vi "KeyboardController.vi"(8 "Manual Control Cluster":T1 {"Speed" scale=0.0..5.0}) -> (0 "Manual Control Cluster":T1 {"Speed" scale=0.0..5.0}, 1 "Extend":bool, 2 "Stop Button":bool, 3 "Retract":bool, 4 "Speed":dbl)   [LabVIEW 2021]
uses:
  <vilib>/event_ctls.llb/eventvkey.ctl
  <vilib>/event_ctls.llb/lveventtype.ctl
  <vilib>/event_ctls.llb/eventsource.ctl
  ManualConttrolCluster.ctl
panel:
  out "ScanCode":i16
  out "Time":u32
  out "PlatMods":T2
  out "Mods":cluster{"Num Pad":bool, "Menu Key":bool}
  out "Source":T3 items=["LabVIEW UI"=0, "ActiveX"=1, "User Event"=25]
  out "Type":T4=enum."Value Change"
  out "VKey":T5
  out "Char":i16
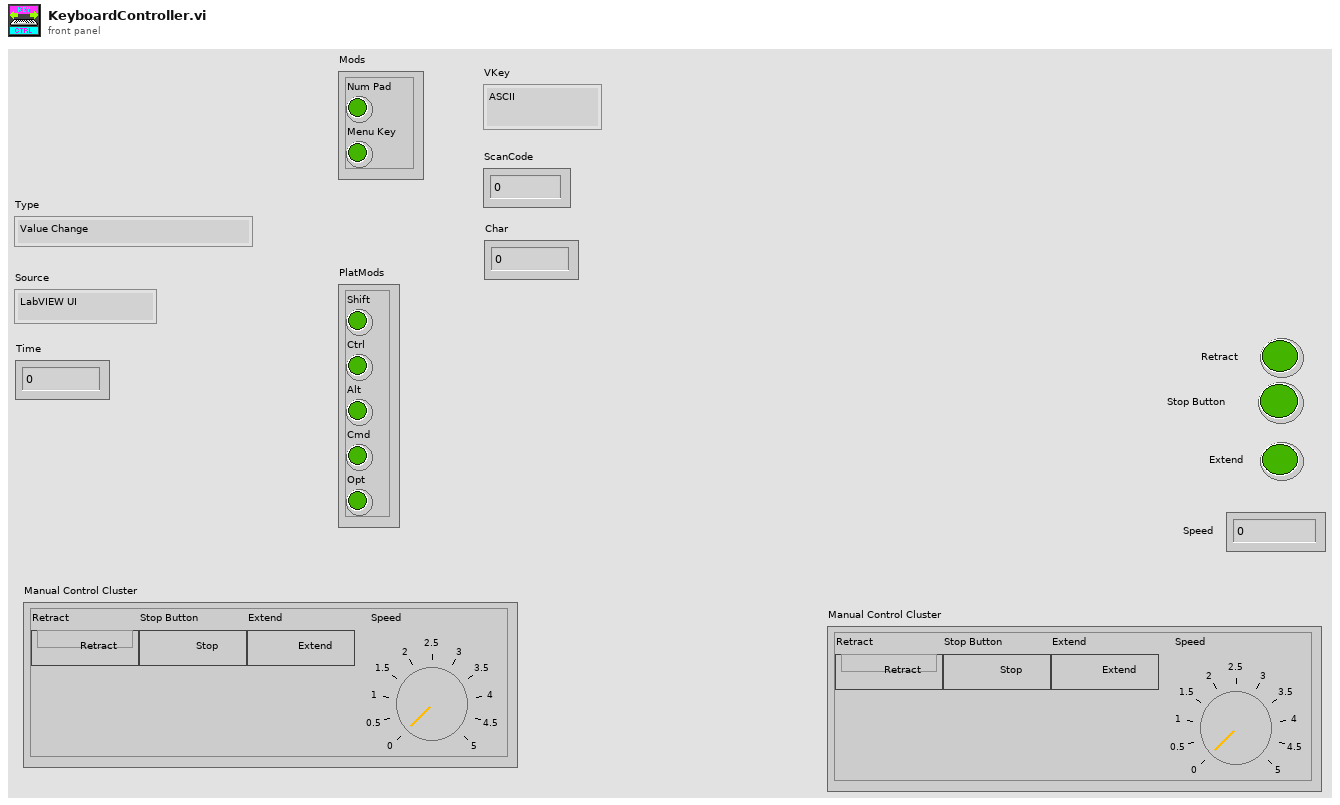
[diagram p1: front panel]
types:
  T1 = typedef "ManualConttrolCluster.ctl" = cluster{"Retract":bool, "Stop Button":bool, "Extend":bool, "Speed":dbl}
  T2 = cluster{"Shift":bool, "Ctrl":bool, "Alt":bool, "Cmd":bool, "Opt":bool}
  T3 = typedef "eventsource.ctl" = u32
  T4 = typedef "lveventtype.ctl" = enum32{"Null", "Timeout", "Annotation Menu Selection", "Annotation Menu Selection?", "App Instance Close", "App Instance Close?", "Autoscale Range Change", "Bookmark Info Change", "Cell Edit", "Cell Edit?", "Cursor Grab", "Cursor Grab?", "Cursor Menu Selection", "Cursor Menu Selection?", "Cursor Move", "Cursor Release", "Data Change", "Direction Change", "Display State Change", "Drag Ended", "Drag Enter", "Drag Leave", "Drag Over", "Drag Source Update", "Drag Starting", "Drag Starting?", "Drop", "Exec State Change", "Key Down", "Key Down?", "Key Repeat", "Key Repeat?", "Key Up", "Listbox Double Click", "Menu Activation?", "Menu Selection (App)", "Menu Selection? (App)", "Menu Selection (User)", "Mouse Down", "Mouse Down?", "Mouse Enter", "Mouse Leave", "Mouse Move", "Mouse Up", "Mouse Wheel", "NI Security User Change (App)", "Pane Size", "Panel Close", "Panel Close?", "Panel Resize", "Plot Attribute Change", "Scale Range Change", "Shortcut Menu Activation?", "Shortcut Menu Selection (App)", "Shortcut Menu Selection? (App)", "Shortcut Menu Selection (User)", "Tree Double Click", "Tree Drag", "Tree Drag?", "Tree Drop", "Tree Drop?", "Tree Item Close", "Tree Item Close?", "Tree Item Open", "Tree Item Open?", "User Event", "Value Change"}
  T5 = typedef "eventvkey.ctl" = enum16{"ASCII", "Enter", "Return", "Shift", "Ctrl", "Alt", "Cmd", "Opt", "Caps", "NumLock", "Clear", "Break", "Up", "Down", "Left", "Right", "Insert", "Delete", "Home", "End", "PageUp", "PageDown", "Escape", "Help", "Pause", "ScrollLock", "F1", "F2", "F3", "F4", "F5", "F6", "F7", "F8", "F9", "F10", "F11", "F12", "F13", "F14", "F15", "F16", "F17", "F18", "F19", "F20", "F21", "F22", "F23", "F24", "Play", "VolumeUp", "VolumeDown", "Mute", "Two Byte Char"}
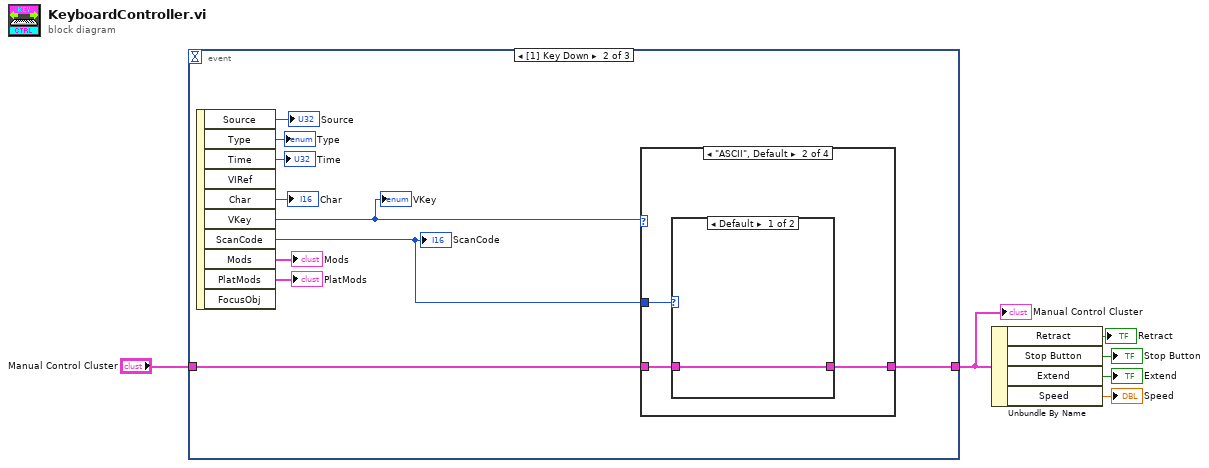
[diagram p0: block diagram]
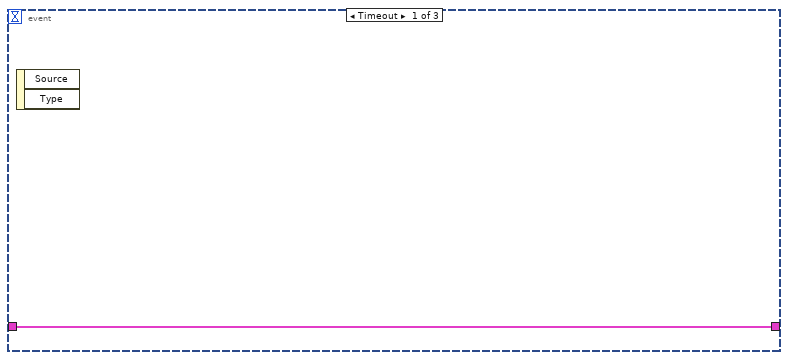
[diagram p2: hidden frame]
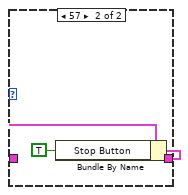
[diagram p4: hidden frame]
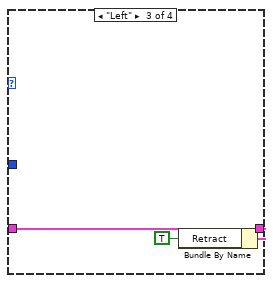
[diagram p5: hidden frame]
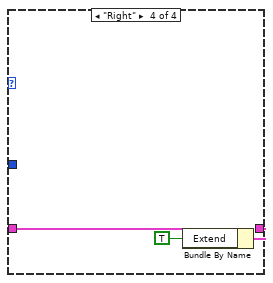
[diagram p6: hidden frame]
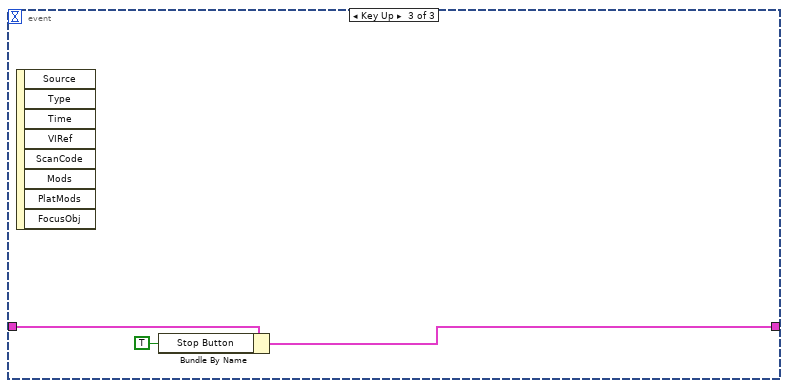
[diagram p7: hidden frame]
diagram:
  n1 = event shown="[1] Key Down" {
    selector: _ -> [_ _ _]
    dyn-events: _ -> [_ _ _]
    timeout: _ -> [_ _ _]
    tunnel: [w7 w9 w33] -> w2
    tunnel: "Manual Control Cluster" -> [w7 w8 w34]
    event Timeout {
      n2 = event-data() -> ()  [unwired: 1 in, 2 out]
    }
    event Key Down {
      n3 = event-data() -> ("Source"=→"Source":T3, "Type"=→"Type":T4, "Time"=→"Time":u32, "Char"=→"Char":i16, "VKey"=w11:T5, "ScanCode"=w10:i16, "Mods"=→"Mods":cluster{"Num Pad":bool, "Menu Key":bool}, "PlatMods"=→"PlatMods":T2)  [unwired: 1 in, 2 out]
      "VKey" <- w11
      "ScanCode" <- w10
      n4 = case shown="\"ASCII\", Default" w11 {
        tunnel: w10 -> [_ w21 _ _]
        tunnel: [w18 w20 w27 w30] -> w9
        tunnel: w8 -> [w18 w19 w28 w31]
        frame "Enter" {
        }
        frame "ASCII", Default {
          n5 = case shown="Default" w21 {
            tunnel: [w22 w25] -> w20
            tunnel: w19 -> [w22 w24]
            frame Default {
            }
            frame 57 {
              n6 = Bundle By Name(cluster=w24, "Stop Button"=TRUE) -> (w25:T1)
            }
          }
        }
        frame "Left" {
          n7 = Bundle By Name(cluster=w28, "Retract"=TRUE) -> (w27:T1)
        }
        frame "Right" {
          n8 = Bundle By Name(cluster=w31, "Extend"=TRUE ("Retract")) -> (w30:T1)
        }
      }
    }
    event Key Up {
      n9 = event-data() -> ()  [unwired: 1 in, 8 out]
      n10 = Bundle By Name(cluster=w34, "Stop Button"=TRUE) -> (w33:T1)
    }
  }
  "Manual Control Cluster" <- w2
  n11 = Unbundle By Name(w2) -> ("Retract"=→"Retract":bool, "Stop Button"=→"Stop Button":bool, "Extend"=→"Extend":bool, "Speed"=→"Speed":dbl)
